vi "CS++CoreContent-Linux.vi"() -> (0 "CS++Classes & Messages":T1(array[cluster]))   [LabVIEW 2015]
doc: "Place actor and class constants that should be included included in an application on the blockdiagramm."
uses:
  <vilib>/ActorFramework/Message/Message.lvclass
  Actors/CS++StartActor/CS++StartActor.lvclass
  Actors/CS++PVMonitor/CS++PVMonitor.lvclass
  Actors/CS++PVProxy/CS++PVProxy.lvclass
  Actors/CS++DeviceActor/CS++DeviceActor.lvclass
  Classes/CS++BaseClasses/Base/CS++Base.lvclass
  Classes/CS++BaseClasses/Factory/CS++Factory.lvclass
  Classes/CS++BaseClasses/Reference/CS++Reference.lvclass
  Classes/CS++ProcessVariables/ProcessVariable/PV.lvclass
  Classes/CS++ProcessVariables/PVConnection/PVConnection.lvclass
  Classes/CS++BaseClasses/MessageLogger/CS++MessageLogger.lvclass
  Classes/CS++ProcessVariables/DSConnection/DSConnection.lvclass
  Actors/CS++DSMonitor/CS++DSMonitor.lvclass
  Actors/CS++BaseActor/CS++BaseActor.lvclass
panel:
  # "Place actor and class constants on the blockdiagramm."
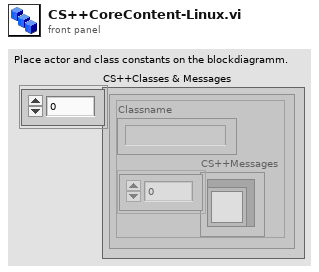
[diagram p1: front panel]
types:
  T1 = cluster{"Classname":string, "CS++Messages":refnum<class "Message.lvclass">[]}[]
  T2 = cluster{"class name":string, "CS++Messages":refnum<class "Message.lvclass">[]}
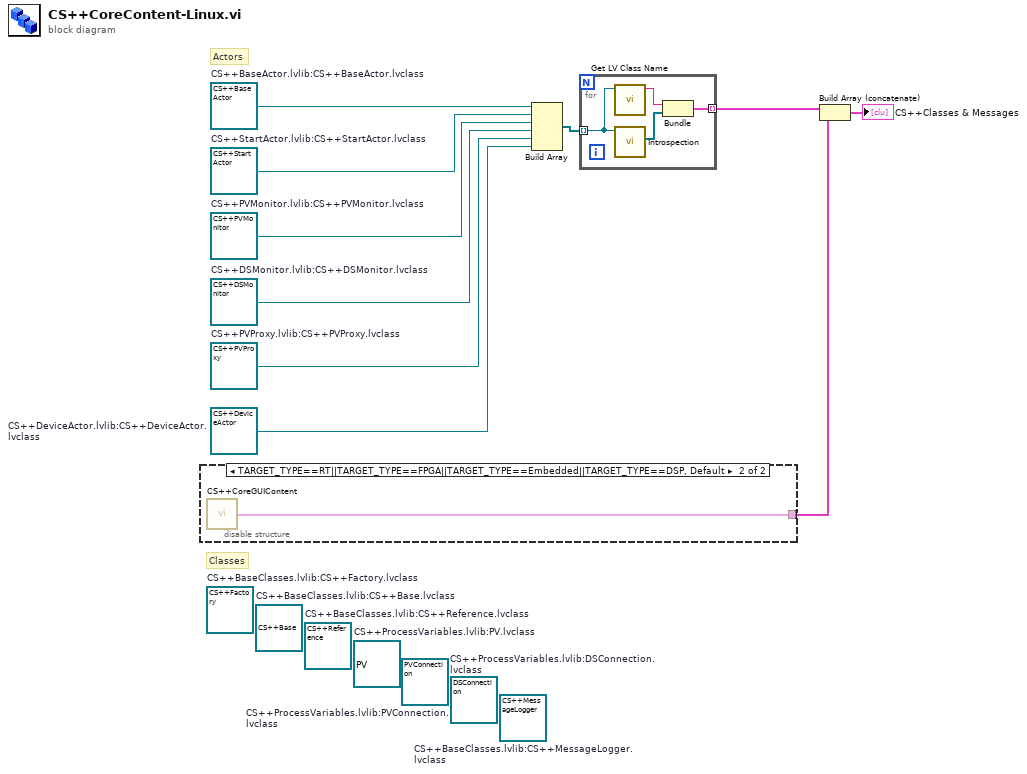
[diagram p0: block diagram]
diagram:
  w1 = refnum<class "CS++BaseActor.lvclass"> refnum  # CS++BaseActor.lvlib:CS++BaseActor.lvclass
  w2 = refnum<class "CS++DSMonitor.lvclass"> refnum  # CS++DSMonitor.lvlib:CS++DSMonitor.lvclass
  (unwired) refnum<class "DSConnection.lvclass"> refnum  # CS++ProcessVariables.lvlib:DSConnection.lvclass
  (unwired) refnum<class "CS++MessageLogger.lvclass"> refnum  # CS++BaseClasses.lvlib:CS++MessageLogger.lvclass
  (unwired) refnum<class "PVConnection.lvclass"> refnum  # CS++ProcessVariables.lvlib:PVConnection.lvclass
  (unwired) refnum<class "PV.lvclass"> refnum  # CS++ProcessVariables.lvlib:PV.lvclass
  (unwired) refnum<class "CS++Reference.lvclass"> refnum  # CS++BaseClasses.lvlib:CS++Reference.lvclass
  (unwired) refnum<class "CS++Factory.lvclass"> refnum  # CS++BaseClasses.lvlib:CS++Factory.lvclass
  (unwired) refnum<class "CS++Base.lvclass"> refnum  # CS++BaseClasses.lvlib:CS++Base.lvclass
  w6 = refnum<class "CS++DeviceActor.lvclass"> refnum  # CS++DeviceActor.lvlib:CS++DeviceActor.lvclass
  w7 = refnum<class "CS++PVProxy.lvclass"> refnum  # CS++PVProxy.lvlib:CS++PVProxy.lvclass
  w8 = refnum<class "CS++PVMonitor.lvclass"> refnum  # CS++PVMonitor.lvlib:CS++PVMonitor.lvclass
  w9 = refnum<class "CS++StartActor.lvclass"> refnum  # CS++StartActor.lvlib:CS++StartActor.lvclass
  # "Classes"
  # "Actors"
  n1 = disable-structure shown="TARGET_TYPE==RT||TARGET_TYPE==FPGA||TARGET_TYPE==Embedded||TARGET_TYPE==DSP, Default" {
    disable-tunnel: [_ w11] -> w5
    frame condition #0 (active) {
    }
    frame condition #1 {
      n2 = call "CS++CoreGUIContent.vi"() -> ("CS++Classes & Messages"=w11:T1)  [unwired: 1 in]
    }
  }
  n3 = Build Array(w1, w9, w8, w2, w7, w6) -> (w10:refnum<class "CS++BaseActor.lvclass">[])
  n4 = for {
    tunnel: w10 -> [w15] mode=indexing
    tunnel: [w12] -> w3 mode=indexing
    n5 = call <vilib>:"Get LV Class Name.vi"("object"=w15) -> ("class name"=w14:string)  [unwired: 9 in, 1 out]
    n6 = call "Introspection.vi"("CS++BaseActor in"=w15) -> ("CS++Messages"=w13:refnum<class "Message.lvclass">[])  [unwired: 8 in, 2 out]
    n7 = Bundle("class name"=w14, "CS++Messages"=w13) -> (w12:T2)  [unwired: 1 in]
  }
  n8 = Build Array (concatenate)(w3, w5) -> (→"CS++Classes & Messages":T1)
